vi "Super Market Billing System edit 3.1.vi"() -> ()   [LabVIEW 2021]
uses:
  <vilib>/Utility/file.llb/Write Delimited Spreadsheet (DBL).vi
panel:
  in  "Tab Control":enum32{"Page 1", "Page 2"}(tab)
  out "Horizontal Progress Bar":u8(slide) scale=0.0..100.0
  in  "Refresh Button":bool
  in  "Password":string
  in  "System Login":string
  in  "file path (dialog if empty) 2":path
  in  "stop":bool
  in  "Rise 5Kg":bool
  in  "Dal 1Kg":bool
  in  "Salt 400g":bool
  in  "Coconut Oil 1L":bool
  in  "Cilli Powder 100g":bool
  in  "Curry Powder 100g":bool
  in  "Turmeric Powder 50g":bool
  in  "Milk Powder 1kg":bool
  in  "Sugar  1kg":bool
  out "Rs.":dbl
  out "Rs.":dbl
  out "Rs.":dbl
  out "Rs.":dbl
  in  "quantity 14":dbl
  out "Rs.":dbl
  in  "quantity 15":dbl
  out "Rs":dbl
  in  "quantity 16":dbl
  out "Rs.":dbl
  in  "quantity 13":dbl
  in  "Quantities 4":dbl
  in  "quantity 12":dbl
  in  "quantity 11":dbl
  in  "quantity 10":dbl
  in  "Tea 100g":bool
  in  "Quantities":dbl
  in  "quantity 17":dbl
  out "Rs.":dbl
  out "Rs.":dbl
  out "Rs.":dbl
  out "Rs.":dbl
  out "Rs.":dbl
  out "Rs.":dbl
  out "Rs.":dbl
  out "Rs. 5":dbl
  out "Rs. 6":dbl
  out "Rs.":dbl
  out "Rs.":dbl
  out "Rs.":dbl
  out "Rs.":dbl
  out "Discount   Rs.":dbl
  in  "kg":dbl
  in  "Papaya":bool
  in  "kg":dbl
  in  "Graps":bool
  in  "kg":dbl
  in  "Orange":bool
  in  "kg":dbl
  in  "Apple":bool
  in  "kg":dbl
  in  "Banana":bool
  out "Bill   Rs.":dbl
  out "Discount percentage":string
  out "Total Bill   Rs.":dbl
  in  "kg":dbl
  in  "Cabege":bool
  in  "kg":dbl
  in  "Bringle":bool
  in  "kg":dbl
  in  "Beans":bool
  in  "kg":dbl
  in  "Leeks":bool
  in  "kg":dbl
  in  "Carrot":bool
  # "WELCOME TO A SUPER MARCKET...."
  # "Price per 1kg (Rs.)"
  # "Quantities(kg)"
  # "Price  (Rs.)"
  # "Quantities"
  # "Vegetables"
  # "Product List"
  # "Fruits"
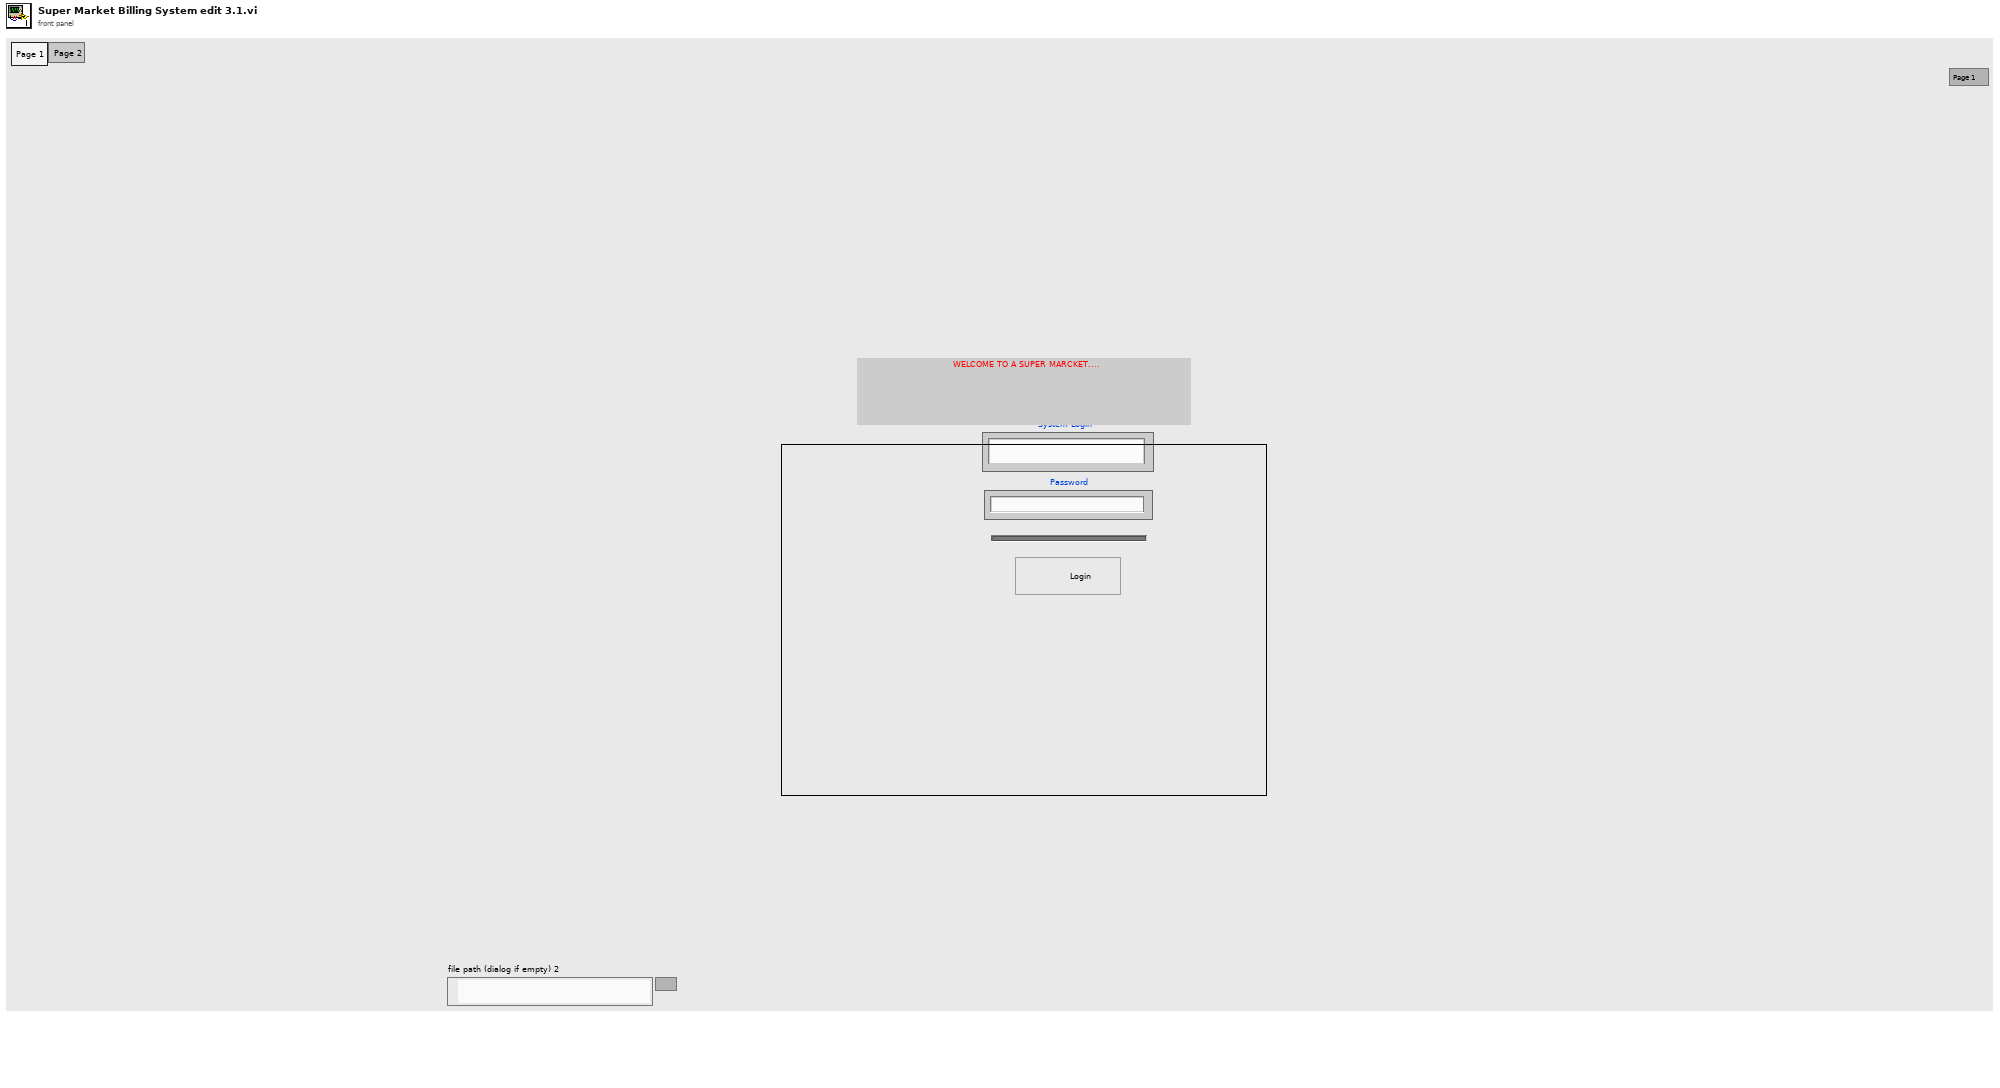
[diagram p1: front panel]
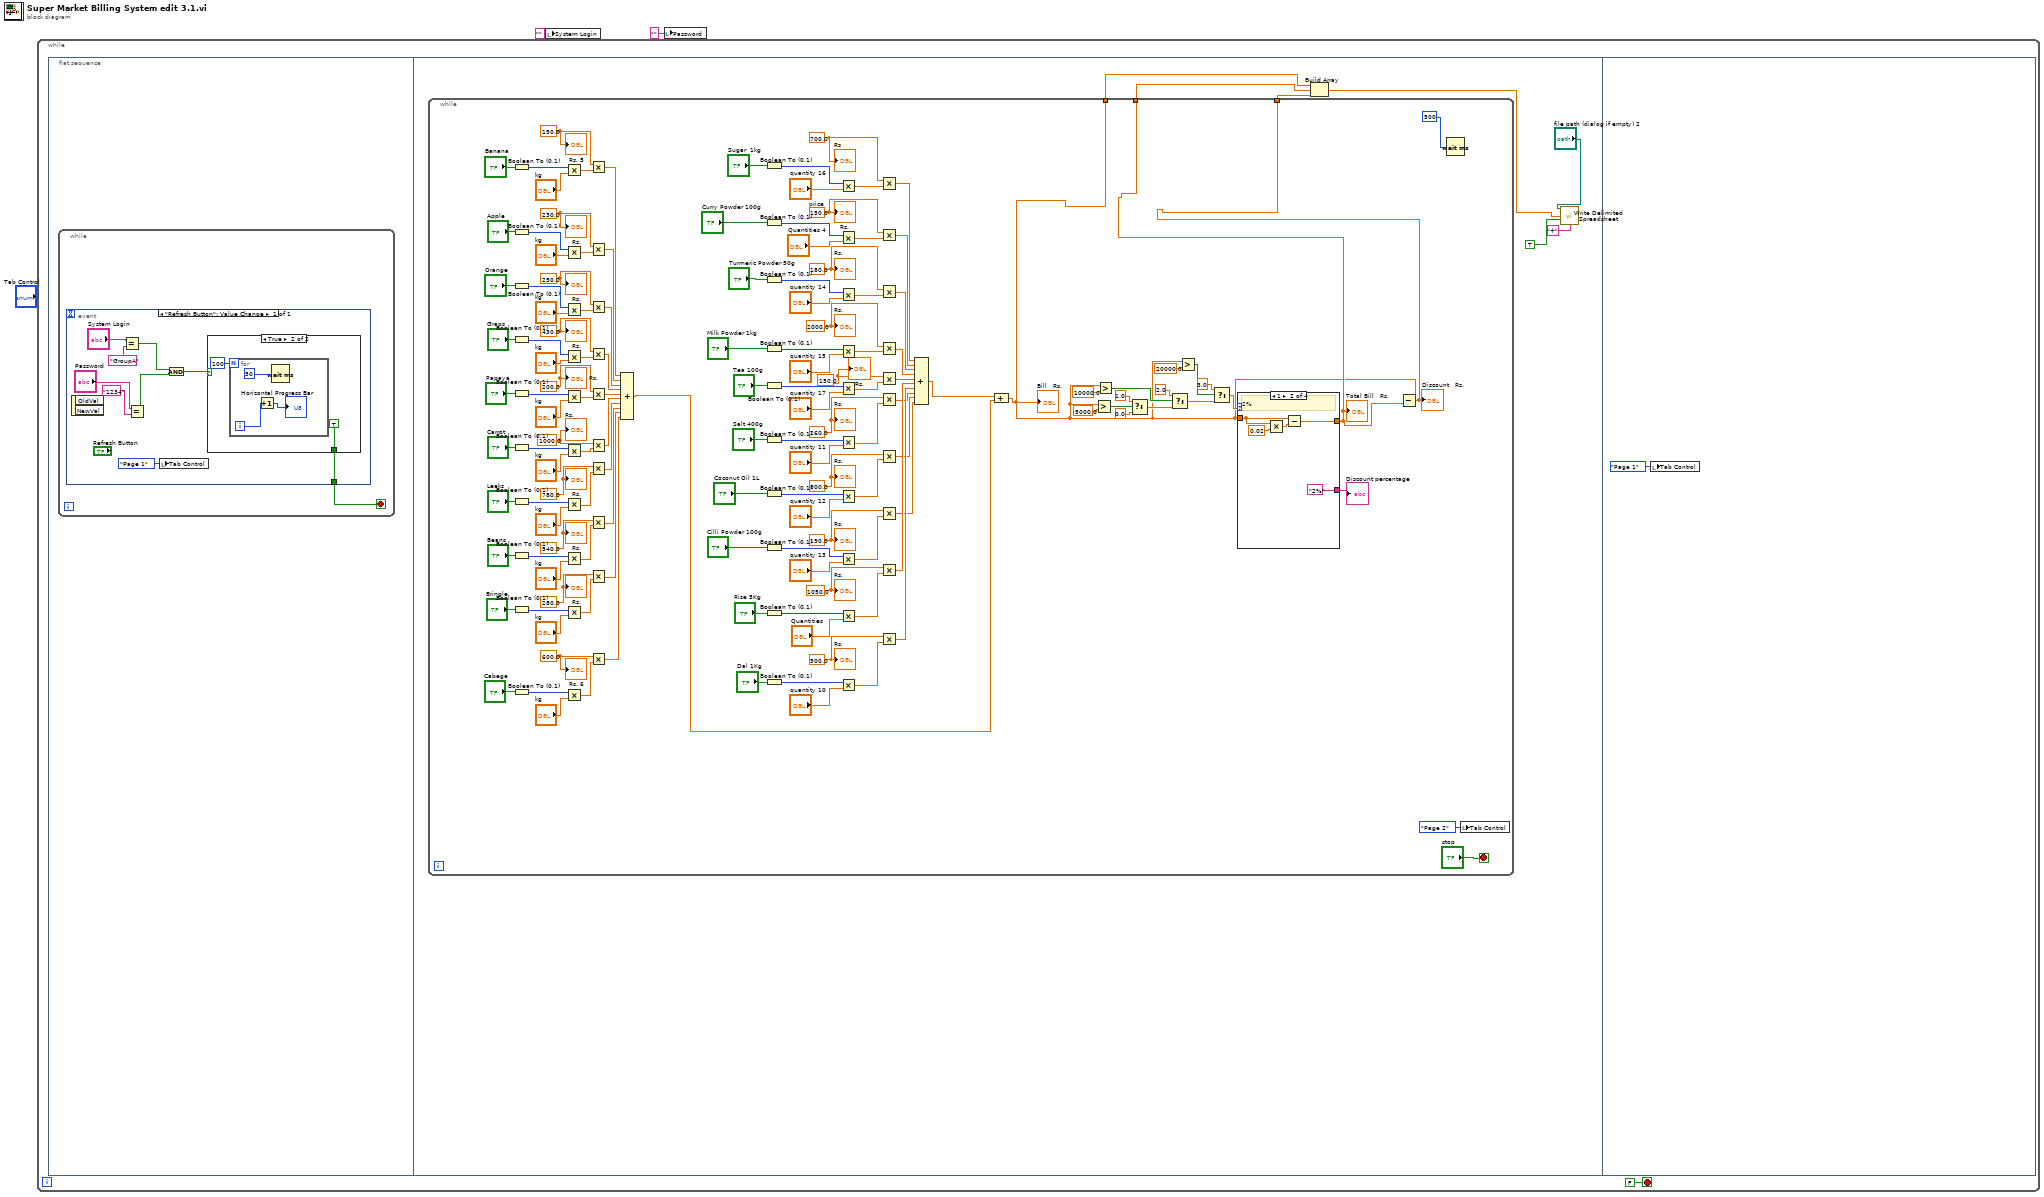
[diagram p0: block diagram]
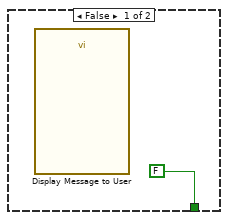
[diagram p2: hidden frame]
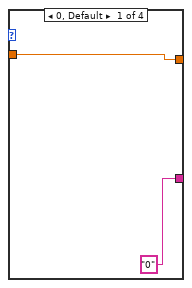
[diagram p3: hidden frame]
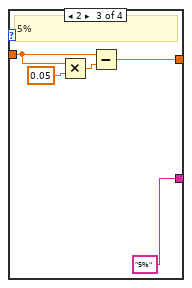
[diagram p4: hidden frame]
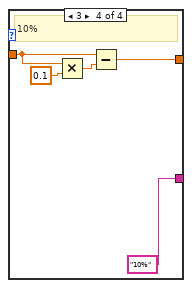
[diagram p5: hidden frame]
diagram:
  n1 = while {
    stop <- FALSE stop-if-true
    n2 = flat-sequence {
      frame #0 {
        n3 = while {
          stop <- w4 stop-if-true
          n4 = event shown="[0] \"Refresh Button\": Value Change" {
            selector: _ -> [_]
            dyn-events: _ -> [_]
            timeout: _ -> [_]
            tunnel: [w7] -> w4
            event "Refresh Button": Value Change {
              n5 = event-data() -> ()  [unwired: 1 in, 2 out]
              n6 = Equal?(x="System Login", y="GroupA") -> (x = y?=w10:bool)
              n7 = Equal?(x="Password", y="1234") -> (x = y?=w9:bool)
              n8 = local write "Tab Control"(enum32{"Page 1", "Page 2"}."Page 1" ("Tab Control")) -> ()
              n9 = And(x=w10, y=w9) -> (x .and. y?=w8:bool)
              n10 = case shown="True" w8 {
                tunnel: [FALSE TRUE] -> w7
                frame False {
                  n11 = call "Display Message to User"() -> ()  [unwired: 10 in, 2 out]
                }
                frame True {
                  n12 = for {
                    N: 100 -> [_]
                    i -> [w17]
                    n13 = Increment(x=w17) -> (x+1=→"Horizontal Progress Bar":i32)
                    n14 = Wait (ms)(milliseconds to wait=u32 50 ("millisecond timer value")) -> ()  [unwired: 1 out]
                  }
                }
              }
            }
          }
        }
      }
      frame #1 {
        n15 = while {
          tunnel: [w27] -> w26
          tunnel: [w28] -> w25
          tunnel: [w29] -> w24
          stop <- "stop" stop-if-true
          w55 = 200.0 ("price")
          w48 = 430.0 ("price")
          w45 = 250.0 ("price")
          w38 = 230.0 ("price")
          w35 = 150.0 ("price")
          w80 = 600.0 ("price")
          w73 = 280.0 ("price")
          w70 = 540.0 ("price")
          w63 = 780.0 ("price")
          w60 = 1000.0 ("price")
          w141 = 150.0 ("price")
          w134 = 700.0 ("price")
          w131 = 2000.0 ("price")
          w124 = 180.0 ("price")
          w121 = 150.0  # price
          w166 = 190.0 ("price")
          w159 = 800.0 ("price")
          w156 = 260.0 ("price")
          w149 = 500.0 ("price")
          w146 = 1050.0 ("price")
          n16 = Boolean To (0,1)(Boolean="Banana") -> (0, 1=w33:i16)
          n17 = Boolean To (0,1)(Boolean="Apple") -> (0, 1=w40:i16)
          n18 = Boolean To (0,1)(Boolean="Orange") -> (0, 1=w43:i16)
          n19 = Boolean To (0,1)(Boolean="Graps") -> (0, 1=w50:i16)
          n20 = Boolean To (0,1)(Boolean="Papaya") -> (0, 1=w53:i16)
          n21 = Boolean To (0,1)(Boolean="Carrot") -> (0, 1=w58:i16)
          n22 = Boolean To (0,1)(Boolean="Leeks") -> (0, 1=w65:i16)
          n23 = Boolean To (0,1)(Boolean="Beans") -> (0, 1=w68:i16)
          n24 = Boolean To (0,1)(Boolean="Bringle") -> (0, 1=w75:i16)
          n25 = Boolean To (0,1)(Boolean="Cabege") -> (0, 1=w78:i16)
          n26 = Multiply(x=w33, y="kg") -> (x*y=w36:dbl)
          n27 = Multiply(x=w40, y="kg") -> (x*y=w37:dbl)
          n28 = Multiply(x=w43, y="kg") -> (x*y=w46:dbl)
          n29 = Multiply(x=w50, y="kg") -> (x*y=w47:dbl)
          n30 = Multiply(x=w53, y="kg") -> (x*y=w56:dbl)
          n31 = Multiply(x=w58, y="kg") -> (x*y=w61:dbl)
          n32 = Multiply(x=w65, y="kg") -> (x*y=w62:dbl)
          n33 = Multiply(x=w68, y="kg") -> (x*y=w71:dbl)
          n34 = Multiply(x=w75, y="kg") -> (x*y=w72:dbl)
          n35 = Multiply(x=w78, y="kg") -> (x*y=w81:dbl)
          n36 = Multiply(x=w35, y=w36) -> (x*y=w96:dbl)
          n37 = Multiply(x=w38, y=w37) -> (x*y=w97:dbl)
          n38 = Multiply(x=w45, y=w46) -> (x*y=w98:dbl)
          n39 = Multiply(x=w48, y=w47) -> (x*y=w99:dbl)
          n40 = Multiply(x=w55, y=w56) -> (x*y=w100:dbl)
          n41 = Multiply(x=w60, y=w61) -> (x*y=w101:dbl)
          n42 = Multiply(x=w63, y=w62) -> (x*y=w102:dbl)
          n43 = Multiply(x=w70, y=w71) -> (x*y=w103:dbl)
          n44 = Multiply(x=w73, y=w72) -> (x*y=w104:dbl)
          n45 = Multiply(x=w80, y=w81) -> (x*y=w105:dbl)
          n46 = Compound Arithmetic op=ADD(w96, w97, w98, w99, w100, w101, w102, w103, w104, w105) -> (w30:dbl)
          n47 = Boolean To (0,1)(Boolean="Sugar  1kg") -> (0, 1=w136:i16)
          n48 = Boolean To (0,1)(Boolean="Curry Powder 100g") -> (0, 1=w119:i16)
          n49 = Boolean To (0,1)(Boolean="Turmeric Powder 50g") -> (0, 1=w126:i16)
          n50 = Boolean To (0,1)(Boolean="Milk Powder 1kg") -> (0, 1=w129:i16)
          n51 = Boolean To (0,1)(Boolean="Tea 100g") -> (0, 1=w139:i16)
          n52 = Boolean To (0,1)(Boolean="Salt 400g") -> (0, 1=w154:i16)
          n53 = Boolean To (0,1)(Boolean="Coconut Oil 1L") -> (0, 1=w161:i16)
          n54 = Boolean To (0,1)(Boolean="Cilli Powder 100g") -> (0, 1=w164:i16)
          n55 = Boolean To (0,1)(Boolean="Rise 5Kg") -> (0, 1=w144:i16)
          n56 = Boolean To (0,1)(Boolean="Dal 1Kg") -> (0, 1=w151:i16)
          n57 = Multiply(x=w136, y="quantity 16") -> (x*y=w133:dbl)
          n58 = Multiply(x=w119, y="Quantities 4") -> (x*y=w122:dbl)
          n59 = Multiply(x=w126, y="quantity 14") -> (x*y=w123:dbl)
          n60 = Multiply(x=w129, y="quantity 15") -> (x*y=w132:dbl)
          n61 = Multiply(x=w139, y="quantity 17") -> (x*y=w142:dbl)
          n62 = Multiply(x=w154, y="quantity 11") -> (x*y=w157:dbl)
          n63 = Multiply(x=w161, y="quantity 12") -> (x*y=w158:dbl)
          n64 = Multiply(x=w164, y="quantity 13") -> (x*y=w167:dbl)
          n65 = Multiply(x=w144, y="Quantities") -> (x*y=w147:dbl)
          n66 = Multiply(x=w151, y="quantity 10") -> (x*y=w148:dbl)
          n67 = Multiply(x=w134, y=w133) -> (x*y=w106:dbl)
          n68 = Multiply(x=w121, y=w122) -> (x*y=w115:dbl)
          n69 = Multiply(x=w124, y=w123) -> (x*y=w114:dbl)
          n70 = Multiply(x=w131, y=w132) -> (x*y=w113:dbl)
          n71 = Multiply(x=w141, y=w142) -> (x*y=w112:dbl)
          n72 = Multiply(x=w156, y=w157) -> (x*y=w109:dbl)
          n73 = Multiply(x=w159, y=w158) -> (x*y=w108:dbl)
          n74 = Multiply(x=w166, y=w167) -> (x*y=w107:dbl)
          n75 = Multiply(x=w146, y=w147) -> (x*y=w111:dbl)
          n76 = Multiply(x=w149, y=w148) -> (x*y=w110:dbl)
          n77 = Compound Arithmetic op=ADD(w106, w115, w114, w113, w112, w111, w110, w109, w108, w107) -> (w31:dbl)
          n78 = Compound Arithmetic op=ADD(w31, w30) -> (w27:dbl)
          "Bill   Rs." <- w27
          n79 = Greater?(x=w27, y=5000.0) -> (0:w93:bool)
          n80 = Greater?(x=w27, y=10000.0) -> (0:w94:bool)
          n81 = Select(t=1.0, s=w93, f=0.0) -> (s? t:f=w89:dbl)
          n82 = Select(t=2.0, s=w94, f=w89) -> (s? t:f=w90:dbl)
          n83 = Greater?(x=w27, y=20000.0) -> (0:w95:bool)
          n84 = Select(t=3.0, s=w95, f=w90) -> (s? t:f=w91:dbl)
          n85 = case shown="1" w91 {
            tunnel: [w170 w174 w177 w182] -> w28
            tunnel: w27 -> [w170 w173 w178 w183]
            tunnel: ["0" ("discount") "2%" ("discount") "5%" ("discount") "10%" ("discount")] -> w92
            frame 0, Default {
            }
            frame 1 {
              # "2%"
              n86 = Multiply(x=w173, y=0.02) -> (x*y=w171:dbl)
              n87 = Subtract(x=w173, y=w171) -> (x-y=w174:dbl)
            }
            frame 2 {
              # "5%"
              n88 = Multiply(x=w178, y=0.05) -> (x*y=w179:dbl)
              n89 = Subtract(x=w178, y=w179) -> (x-y=w177:dbl)
            }
            frame 3 {
              # "10%"
              n90 = Multiply(x=w183, y=0.1) -> (x*y=w184:dbl)
              n91 = Subtract(x=w183, y=w184) -> (x-y=w182:dbl)
            }
          }
          "Total Bill   Rs." <- w28
          "Discount percentage" <- w92
          n92 = Subtract(x=w27, y=w28) -> (x-y=w29:dbl)
          "Discount   Rs." <- w29
          n93 = Wait (ms)(milliseconds to wait=u32 500) -> ()  [unwired: 1 out]
          n94 = local write "Tab Control"(enum32{"Page 1", "Page 2"}."Page 2" ("Tab Control")) -> ()
          "Rs." <- w146
          "Rs." <- w149
          "Rs." <- w156
          "Rs." <- w159
          "Rs." <- w166
          "Rs." <- w121
          "Rs." <- w124
          "Rs." <- w131
          "Rs" <- w134
          "Rs." <- w141
          "Rs." <- w60
          "Rs." <- w63
          "Rs." <- w70
          "Rs." <- w73
          "Rs. 6" <- w80
          "Rs. 5" <- w35
          "Rs." <- w38
          "Rs." <- w45
          "Rs." <- w48
          "Rs." <- w55
        }
        n95 = Build Array "Build Array"(w26, w25, w24) -> (w22:dbl[])
        n96 = call-poly <vilib>:"Write Delimited Spreadsheet.vi"("file path (dialog if empty)"="file path (dialog if empty) 2", "1D data"=w22, "append to file? (new file:F)"=TRUE, "delimiter (\\t)"="+" ("delimiter (\\t)")) -> ()  [unwired: 10 in, 2 out]
      }
      frame #2 {
        n97 = local write "Tab Control"(enum32{"Page 1", "Page 2"}."Page 1" ("Tab Control")) -> ()
      }
    }
  }
  n98 = local write "System Login"("" ("User Name")) -> ()
  n99 = local write "Password"("" ("Password")) -> ()
